vi "read_c_string_at_memory_address.vi"(6 "string_length":u64, 8 "error in (no error)":errorcluster, 11 "memory_address":u64) -> (0 "error out":errorcluster, 2 "string":string, 3 "memory_address out":u64)   [LabVIEW 2020, in "reqwest.lvlib"]
uses:
  reqwest.lvlib
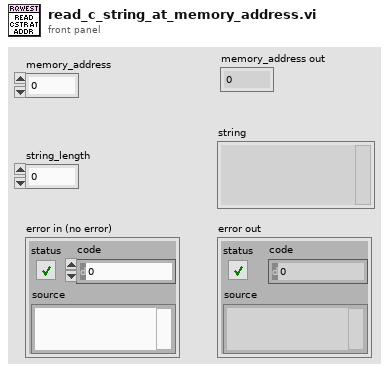
[diagram p1: front panel]
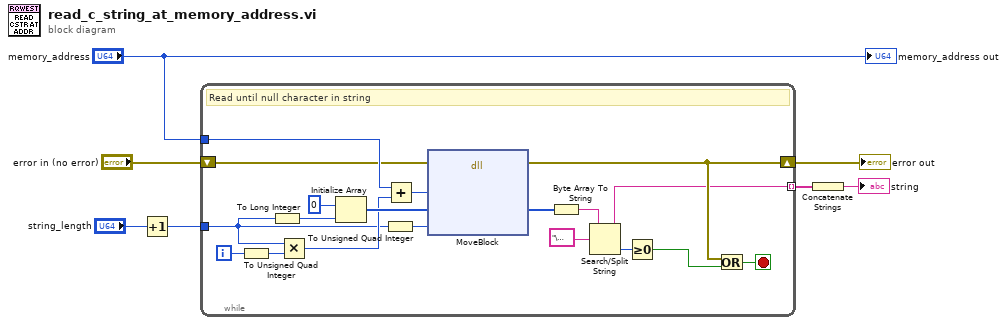
[diagram p0: block diagram]
diagram:
  n1 = Increment(x="string_length") -> (x+1=w1:u64)
  n2 = while {
    tunnel: "memory_address" -> [w25]
    shift-right: [w17] -> w6
    shift-left: "error in (no error)" -> [w24]
    tunnel: [w11] -> w4 mode=indexing
    tunnel: w1 -> [w9]
    i -> [w10]
    stop <- w18 stop-if-true
    # "Read until null character in string"
    n3 = To Unsigned Quad Integer(1:w10) -> (0:w8:u64)
    n4 = To Long Integer(number=w9) -> (32bit integer=w21:i32)
    n5 = Multiply(x=w9, y=w8) -> (x*y=w19:u64)
    n6 = Initialize Array(u8 0, w21) -> (w22:u8[])
    n7 = To Unsigned Quad Integer(1:w9) -> (0:w20:u64)
    n8 = Add(x=w25, y=w19) -> (x+y=w26:u64)
    n9 = dll-call lib="LabVIEW" fn="MoveBlock"(error in=w24, "src"=w26, "dst"=w22, "size"=w20) -> (error out=w17:errorcluster, "dst"=w12:u8[])  [unwired: 5 in, 1 out]
    n10 = Byte Array To String(unsigned byte array=w12) -> (string=w15:string)
    n11 = Search/Split String(string=w15, search string/char (-)="\u0000" ("string")) -> (substring before match=w11:string, offset of match=w14:i32)  [unwired: 1 in, 1 out]
    n12 = Greater Or Equal To 0?(x=w14) -> (x >= 0?=w13:bool)
    n13 = Or(x=w17, y=w13) -> (x .or. y?=w18:bool)
  }
  "error out" <- w6
  n14 = Concatenate Strings(w4) -> (→"string":string)
  "memory_address out" <- "memory_address"
